vi "Teardown.vi"(11 "Ex Event Actor in":refnum<class "Ex Event Actor.lvclass">) -> (3 "Ex Event Actor out":refnum<class "Ex Event Actor.lvclass">)   [LabVIEW 2021, in "Ex Event Actor.lvlib" / "Ex Event Actor.lvclass"]
uses:
  Ex Event Actor.lvclass
  Ex Event Actor.lvclass/Ex Event Actor.ctl
  C:/git/jettl/src/Example/Ex Event Actor/Ex Event Actor/Ex Event Actor.lvclass
  C:/git/jettl/src/Example/String Indicator Event/String Indicator/String Indicator.lvclass
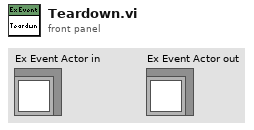
[diagram p1: front panel]
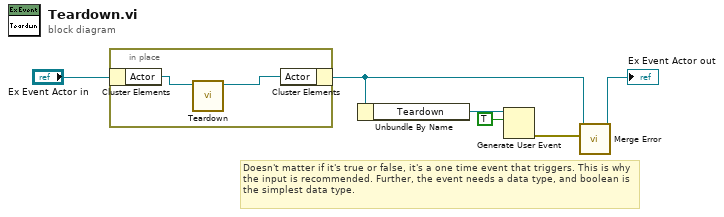
[diagram p0: block diagram]
diagram:
  # "Doesn't matter if it's true or false, it's a one time event that triggers. This is why the input is recommended. Further, the event needs a data type, and boolean is the simplest data type."
  n1 = in-place {
    n2 = in-place-cluster #1("Ex Event Actor in") -> ("Actor"=w8:refnum<class "Actor.lvclass">)
    n3 = call-dynamic "Teardown.vi"("Ex Event Actor in"=w8) -> ("Ex Event Actor out"=w7:refnum<class "Ex Event Actor.lvclass">)  [unwired: 10 in]
    n4 = in-place-cluster #1("Actor"=w7) -> (w3:refnum<class "Ex Event Actor.lvclass">)
  }
  n5 = Unbundle By Name(w3) -> ("Teardown"=w4:refnum<user-event>)
  n6 = Generate User Event(user event=w4, event data cluster=TRUE ("event data")) -> (error out=w1:errorcluster)  [unwired: 2 in, 1 out]
  n7 = call-dynamic "Merge Error.vi"("Error"=w1, "Ex Event Actor in"=w3) -> ("Ex Event Actor out"=→"Ex Event Actor out":refnum<class "Ex Event Actor.lvclass">)  [unwired: 9 in]
